vi "SubVi Json Send.vi"(8 "error in (no error)":errorcluster, 10 "Cluster":T1, 11 "input cluster":T2) -> (0 "error out":errorcluster, 3 "String":string)   [LabVIEW 2015]
uses:
  <vilib>/LVH/i3 JSON/JSON Generation/Add Object Parameter Files/Add Object Parameter - String.vi
  <vilib>/LVH/i3 JSON/i3-json.lvlib
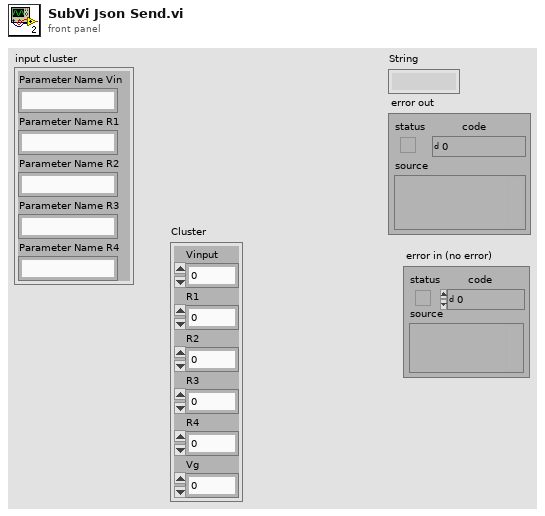
[diagram p1: front panel]
types:
  T1 = cluster{"Vinput":dbl, "R1":dbl, "R2":dbl, "R3":dbl, "R4":dbl, "Vg":dbl}
  T2 = cluster{"Parameter Name Vin":string, "Parameter Name R1":string, "Parameter Name R2":string, "Parameter Name R3":string, "Parameter Name R4":string}
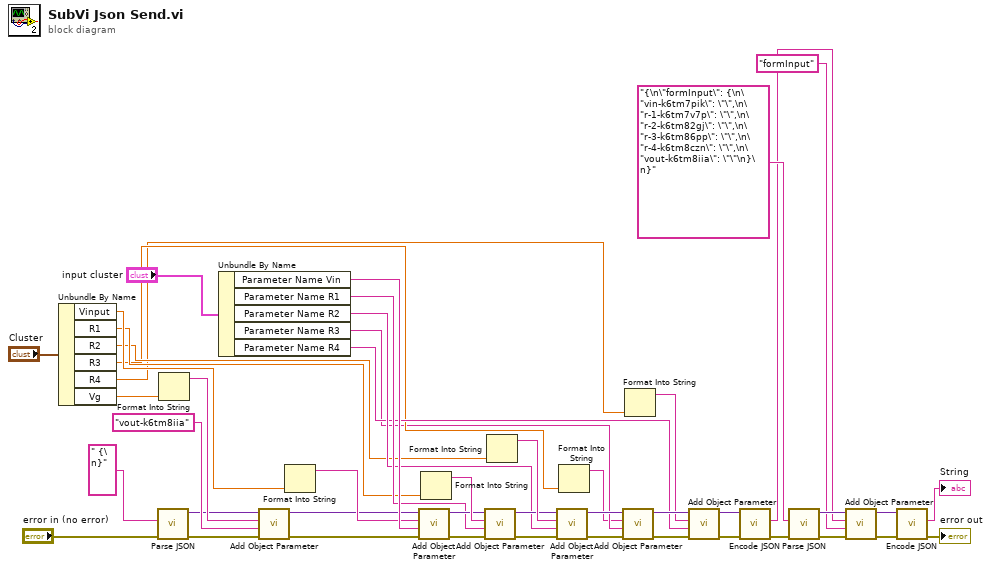
[diagram p0: block diagram]
diagram:
  n1 = Unbundle By Name("Cluster") -> ("Vinput"=w10:dbl, "R1"=w9:dbl, "R2"=w8:dbl, "R3"=w7:dbl, "R4"=w5:dbl, "Vg"=w6:dbl)
  n2 = call <vilib>:"Parse JSON.vi"("error in (no error)"="error in (no error)", "JSON String"=" {\n}" ("String")) -> ("error out"=w3:errorcluster, "JSON Tree"=w40:variant)  [unwired: 6 in, 2 out]
  n3 = Format Into String(w6) -> (resulting string=w41:string)  [unwired: 3 in, 1 out]
  n4 = Unbundle By Name("input cluster") -> ("Parameter Name Vin"=w45:string, "Parameter Name R1"=w36:string, "Parameter Name R2"=w33:string, "Parameter Name R3"=w2:string, "Parameter Name R4"=w30:string)
  n5 = call-poly <vilib>:"Add Object Parameter.vi"("error in (no error)"=w3, "Name"="vout-k6tm8iia", "String"=w41, "JSON Tree in (JSON Object)"=w40) -> ("error out"=w4:errorcluster, "JSON Tree out (JSON Object)"=w39:variant)  [unwired: 6 in]
  n6 = Format Into String(w10) -> (resulting string=w44:string)  [unwired: 3 in, 1 out]
  n7 = call-poly <vilib>:"Add Object Parameter.vi"("error in (no error)"=w4, "Name"=w45, "String"=w44, "JSON Tree in (JSON Object)"=w39) -> ("error out"=w28:errorcluster, "JSON Tree out (JSON Object)"=w37:variant)  [unwired: 6 in]
  n8 = Format Into String(w9) -> (resulting string=w38:string)  [unwired: 3 in, 1 out]
  n9 = call-poly <vilib>:"Add Object Parameter.vi"("error in (no error)"=w28, "Name"=w36, "String"=w38, "JSON Tree in (JSON Object)"=w37) -> ("error out"=w27:errorcluster, "JSON Tree out (JSON Object)"=w34:variant)  [unwired: 6 in]
  n10 = Format Into String(w8) -> (resulting string=w35:string)  [unwired: 3 in, 1 out]
  n11 = call-poly <vilib>:"Add Object Parameter.vi"("error in (no error)"=w27, "Name"=w33, "String"=w35, "JSON Tree in (JSON Object)"=w34) -> ("error out"=w26:errorcluster, "JSON Tree out (JSON Object)"=w32:variant)  [unwired: 6 in]
  n12 = Format Into String(w7) -> (resulting string=w1:string)  [unwired: 3 in, 1 out]
  n13 = call-poly <vilib>:"Add Object Parameter.vi"("error in (no error)"=w26, "Name"=w2, "String"=w1, "JSON Tree in (JSON Object)"=w32) -> ("error out"=w25:errorcluster, "JSON Tree out (JSON Object)"=w31:variant)  [unwired: 6 in]
  n14 = Format Into String(w5) -> (resulting string=w29:string)  [unwired: 3 in, 1 out]
  n15 = call-poly <vilib>:"Add Object Parameter.vi"("error in (no error)"=w25, "Name"=w30, "String"=w29, "JSON Tree in (JSON Object)"=w31) -> ("error out"=w24:errorcluster, "JSON Tree out (JSON Object)"=w23:variant)  [unwired: 6 in]
  n16 = call <vilib>:"Encode JSON.vi"("error in (no error)"=w24, "JSON Tree"=w23) -> ("error out"=w21:errorcluster, "String"=w12:string)  [unwired: 4 in]
  n17 = call <vilib>:"Parse JSON.vi"("error in (no error)"=w21, "JSON String"="{\n\"formInput\": {\n\"vin-k6tm7pik\": \"\",\n\"r-1-k6tm7v7p\": \"\",\n\"r-2-k6tm82gj\": \"\",\n\"r-3-k6tm86pp\": \"\",\n\"r-4-k6tm8czn\": \"\",\n\"vout-k6tm8iia\": \"\"\n}\n}" ("String")) -> ("error out"=w17:errorcluster, "JSON Tree"=w20:variant)  [unwired: 6 in, 2 out]
  n18 = call-poly <vilib>:"Add Object Parameter.vi"("error in (no error)"=w17, "Name"="formInput", "String"=w12, "JSON Tree in (JSON Object)"=w20) -> ("error out"=w18:errorcluster, "JSON Tree out (JSON Object)"=w19:variant)  [unwired: 6 in]
  n19 = call <vilib>:"Encode JSON.vi"("error in (no error)"=w18, "JSON Tree"=w19) -> ("error out"=→"error out":errorcluster, "String"=→"String":string)  [unwired: 4 in]
